vi "PicoScope6000aExampleRapidBlockBulkOverlapped.vi"() -> ()   [LabVIEW 2010]
uses:
  shared/PicoBuffers.ctl
  <vilib>/Waveform/DWDTOps.llb/DWDT Analog to Digital.vi
  PicoScope6000aLib/PicoScope6000aDigitalChannelSettings.ctl
  PicoScope6000aLib/PicoScope6000aAnalogChannelSettings.ctl
  shared/Buffer and Transfer Settings.ctl
  shared/Acquisition Settings.ctl
  shared/Segment Range.ctl
panel:
  in  "Channels":T1={"Channel A Settings "={"Enabled"=TRUE, "Coupling"=50, "Range"=5, "Analogue Offset"=0.0, "BandWidth"=0}, "Channel B Settings "={"Enabled"=FALSE, "Coupling"=50, "Range"=5, "Analogue Offset"=0.0, "BandWidth"=0}, "Channel C Settings "={"Enabled"=FALSE, "Coupling"=50, "Range"=5, "Analogue Offset"=0.0, "BandWidth"=0}, "Channel D Settings "={"Enabled"=FALSE, "Coupling"=50, "Range"=5, "Analogue Offset"=0.0, "BandWidth"=0}, "Channel E Settings "={"Enabled"=FALSE, "Coupling"=50, "Range"=5, "Analogue Offset"=0.0, "BandWidth"=0}, "Channel F Settings "={"Enabled"=FALSE, "Coupling"=50, "Range"=5, "Analogue Offset"=0.0, "BandWidth"=0}, "Channel G Settings "={"Enabled"=FALSE, "Coupling"=50, "Range"=5, "Analogue Offset"=0.0, "BandWidth"=0}, "Channel H Settings "={"Enabled"=FALSE, "Coupling"=50, "Range"=5, "Analogue Offset"=0.0, "BandWidth"=0}} {"Channel H Settings"."BandWidth" items=["Full"=0, "100kHz"=100000, "20kHz"=200000, "1MHz"=1000000, "20MHz"=20000000, "25MHz"=25000000, "50MHz"=50000000, "200MHz"=200000000, "250MHz"=250000000, "500MHz"=500000000]; "Channel H Settings"."Range" items=["10mV"=0, "20mV"=1, "50mV"=2, "100mV"=3, "200mV"=4, "500mV"=5, "1V"=6, "2V"=7, "5V"=8, "10V"=9, "20V"=10, "50V"=11, "100V"=12, "200V"=13, "x10_Probe_100mV"=32, "x10_Probe_200mV"=33, "x10_Probe_500mV"=34, "x10_Probe_1V"=35, "x10_Probe_2V"=36, "x10_Probe_5V"=37, "x10_Probe_10V"=38, "x10_Probe_20V"=39, "x10_Probe_50V"=40, "x10_Probe_100V"=41, "x10_Probe_200V"=42, "x10_Probe_500V"=43, "CURRENT_CLAMP_60A_2A"=10500, "CURRENT_CLAMP_60A_5A"=10501, "CURRENT_CLAMP_60A_10A"=10502, "CURRENT_CLAMP_60A_20A"=10503, "CURRENT_CLAMP_60A_50A"=10504, "CURRENT_CLAMP_60A_60A"=10505, "CURRENT_CLAMP_60A_V2_0_5A"=10600, "CURRENT_CLAMP_60A_V2_1A"=10601, "CURRENT_CLAMP_60A_V2_2A"=10602, "CURRENT_CLAMP_60A_V2_5A"=10603, "CURRENT_CLAMP_60A_V2_10A"=10604, "CURRENT_CLAMP_60A_V2_20A"=10605, "CURRENT_CLAMP_60A_V2_50A"=10606, "CURRENT_CLAMP_60A_V2_60A"=10607, "RESISTANCE_LEAD_NEG5_TO_20OHM"=7000, "RESISTANCE_LEAD_NEG50_TO_200OHM"=7001, "RESISTANCE_LEAD_NEG500_TO_2KOHM"=7002, "RESISTANCE_LEAD_NEG5K_TO_20KOHM"=7003, "RESISTANCE_LEAD_NEG50K_TO_LEAD_200KOHM"=7004, "RESISTANCE_LEAD_NEG500K_TO_LEAD_2MOHM"=7005, "RESISTANCE_LEAD_DIODE_TEST"=7006, "HT_NEG3_TO_5KV"=8950, "HT_NEG3_TO_10KV"=8951, "HT_NEG5_TO_20KV"=8952, "HT_NEG5_TO_50KV"=8953, "HT_NEG5_TO_100KV"=8954, "HT_NEG3_TO_5KV_INVERTED"=8955, "HT_NEG3_TO_10KV_INVERTED"=8956, "HT_NEG5_TO_20KV_INVERTED"=8957, "HT_NEG5_TO_50KV_INVERTED"=8958, "HT_NEG5_TO_100KV_INVERTED"=8959, "TEMPERATURE_NEG50_TO_150DEGC"=9000, "PRESSURE_SENSOR_-100k-150k_PASCALS"=9100, "PRESSURE_SENSOR_-100k_TO_400k_PASCALS"=9101, "PRESSURE_SENSOR_-200k_TO_800k_PASCALS"=9102, "PRESSURE_SENSOR_-400k_TO_1600k_PASCALS"=9103, "PRESSURE_SENSOR_-400k_TO_3400k_PASCALS"=9104, "PRESSURE_SENSOR_-150k_TO_1350k_PASCALS"=9105]; "Channel H Settings"."Coupling" items=["AC"=0, "DC 1M Ohm"=1, "DC 50 Ohm"=50]; "Channel G Settings"."BandWidth" items=["Full"=0, "100kHz"=100000, "20kHz"=200000, "1MHz"=1000000, "20MHz"=20000000, "25MHz"=25000000, "50MHz"=50000000, "200MHz"=200000000, "250MHz"=250000000, "500MHz"=500000000]; "Channel G Settings"."Range" items=["10mV"=0, "20mV"=1, "50mV"=2, "100mV"=3, "200mV"=4, "500mV"=5, "1V"=6, "2V"=7, "5V"=8, "10V"=9, "20V"=10, "50V"=11, "100V"=12, "200V"=13, "x10_Probe_100mV"=32, "x10_Probe_200mV"=33, "x10_Probe_500mV"=34, "x10_Probe_1V"=35, "x10_Probe_2V"=36, "x10_Probe_5V"=37, "x10_Probe_10V"=38, "x10_Probe_20V"=39, "x10_Probe_50V"=40, "x10_Probe_100V"=41, "x10_Probe_200V"=42, "x10_Probe_500V"=43, "CURRENT_CLAMP_60A_2A"=10500, "CURRENT_CLAMP_60A_5A"=10501, "CURRENT_CLAMP_60A_10A"=10502, "CURRENT_CLAMP_60A_20A"=10503, "CURRENT_CLAMP_60A_50A"=10504, "CURRENT_CLAMP_60A_60A"=10505, "CURRENT_CLAMP_60A_V2_0_5A"=10600, "CURRENT_CLAMP_60A_V2_1A"=10601, "CURRENT_CLAMP_60A_V2_2A"=10602, "CURRENT_CLAMP_60A_V2_5A"=10603, "CURRENT_CLAMP_60A_V2_10A"=10604, "CURRENT_CLAMP_60A_V2_20A"=10605, "CURRENT_CLAMP_60A_V2_50A"=10606, "CURRENT_CLAMP_60A_V2_60A"=10607, "RESISTANCE_LEAD_NEG5_TO_20OHM"=7000, "RESISTANCE_LEAD_NEG50_TO_200OHM"=7001, "RESISTANCE_LEAD_NEG500_TO_2KOHM"=7002, "RESISTANCE_LEAD_NEG5K_TO_20KOHM"=7003, "RESISTANCE_LEAD_NEG50K_TO_LEAD_200KOHM"=7004, "RESISTANCE_LEAD_NEG500K_TO_LEAD_2MOHM"=7005, "RESISTANCE_LEAD_DIODE_TEST"=7006, "HT_NEG3_TO_5KV"=8950, "HT_NEG3_TO_10KV"=8951, "HT_NEG5_TO_20KV"=8952, "HT_NEG5_TO_50KV"=8953, "HT_NEG5_TO_100KV"=8954, "HT_NEG3_TO_5KV_INVERTED"=8955, "HT_NEG3_TO_10KV_INVERTED"=8956, "HT_NEG5_TO_20KV_INVERTED"=8957, "HT_NEG5_TO_50KV_INVERTED"=8958, "HT_NEG5_TO_100KV_INVERTED"=8959, "TEMPERATURE_NEG50_TO_150DEGC"=9000, "PRESSURE_SENSOR_-100k-150k_PASCALS"=9100, "PRESSURE_SENSOR_-100k_TO_400k_PASCALS"=9101, "PRESSURE_SENSOR_-200k_TO_800k_PASCALS"=9102, "PRESSURE_SENSOR_-400k_TO_1600k_PASCALS"=9103, "PRESSURE_SENSOR_-400k_TO_3400k_PASCALS"=9104, "PRESSURE_SENSOR_-150k_TO_1350k_PASCALS"=9105]; "Channel G Settings"."Coupling" items=["AC"=0, "DC 1M Ohm"=1, "DC 50 Ohm"=50]; "Channel F Settings"."BandWidth" items=["Full"=0, "100kHz"=100000, "20kHz"=200000, "1MHz"=1000000, "20MHz"=20000000, "25MHz"=25000000, "50MHz"=50000000, "200MHz"=200000000, "250MHz"=250000000, "500MHz"=500000000]; "Channel F Settings"."Range" items=["10mV"=0, "20mV"=1, "50mV"=2, "100mV"=3, "200mV"=4, "500mV"=5, "1V"=6, "2V"=7, "5V"=8, "10V"=9, "20V"=10, "50V"=11, "100V"=12, "200V"=13, "x10_Probe_100mV"=32, "x10_Probe_200mV"=33, "x10_Probe_500mV"=34, "x10_Probe_1V"=35, "x10_Probe_2V"=36, "x10_Probe_5V"=37, "x10_Probe_10V"=38, "x10_Probe_20V"=39, "x10_Probe_50V"=40, "x10_Probe_100V"=41, "x10_Probe_200V"=42, "x10_Probe_500V"=43, "CURRENT_CLAMP_60A_2A"=10500, "CURRENT_CLAMP_60A_5A"=10501, "CURRENT_CLAMP_60A_10A"=10502, "CURRENT_CLAMP_60A_20A"=10503, "CURRENT_CLAMP_60A_50A"=10504, "CURRENT_CLAMP_60A_60A"=10505, "CURRENT_CLAMP_60A_V2_0_5A"=10600, "CURRENT_CLAMP_60A_V2_1A"=10601, "CURRENT_CLAMP_60A_V2_2A"=10602, "CURRENT_CLAMP_60A_V2_5A"=10603, "CURRENT_CLAMP_60A_V2_10A"=10604, "CURRENT_CLAMP_60A_V2_20A"=10605, "CURRENT_CLAMP_60A_V2_50A"=10606, "CURRENT_CLAMP_60A_V2_60A"=10607, "RESISTANCE_LEAD_NEG5_TO_20OHM"=7000, "RESISTANCE_LEAD_NEG50_TO_200OHM"=7001, "RESISTANCE_LEAD_NEG500_TO_2KOHM"=7002, "RESISTANCE_LEAD_NEG5K_TO_20KOHM"=7003, "RESISTANCE_LEAD_NEG50K_TO_LEAD_200KOHM"=7004, "RESISTANCE_LEAD_NEG500K_TO_LEAD_2MOHM"=7005, "RESISTANCE_LEAD_DIODE_TEST"=7006, "HT_NEG3_TO_5KV"=8950, "HT_NEG3_TO_10KV"=8951, "HT_NEG5_TO_20KV"=8952, "HT_NEG5_TO_50KV"=8953, "HT_NEG5_TO_100KV"=8954, "HT_NEG3_TO_5KV_INVERTED"=8955, "HT_NEG3_TO_10KV_INVERTED"=8956, "HT_NEG5_TO_20KV_INVERTED"=8957, "HT_NEG5_TO_50KV_INVERTED"=8958, "HT_NEG5_TO_100KV_INVERTED"=8959, "TEMPERATURE_NEG50_TO_150DEGC"=9000, "PRESSURE_SENSOR_-100k-150k_PASCALS"=9100, "PRESSURE_SENSOR_-100k_TO_400k_PASCALS"=9101, "PRESSURE_SENSOR_-200k_TO_800k_PASCALS"=9102, "PRESSURE_SENSOR_-400k_TO_1600k_PASCALS"=9103, "PRESSURE_SENSOR_-400k_TO_3400k_PASCALS"=9104, "PRESSURE_SENSOR_-150k_TO_1350k_PASCALS"=9105]; "Channel F Settings"."Coupling" items=["AC"=0, "DC 1M Ohm"=1, "DC 50 Ohm"=50]; "Channel E Settings"."BandWidth" items=["Full"=0, "100kHz"=100000, "20kHz"=200000, "1MHz"=1000000, "20MHz"=20000000, "25MHz"=25000000, "50MHz"=50000000, "200MHz"=200000000, "250MHz"=250000000, "500MHz"=500000000]; "Channel E Settings"."Range" items=["10mV"=0, "20mV"=1, "50mV"=2, "100mV"=3, "200mV"=4, "500mV"=5, "1V"=6, "2V"=7, "5V"=8, "10V"=9, "20V"=10, "50V"=11, "100V"=12, "200V"=13, "x10_Probe_100mV"=32, "x10_Probe_200mV"=33, "x10_Probe_500mV"=34, "x10_Probe_1V"=35, "x10_Probe_2V"=36, "x10_Probe_5V"=37, "x10_Probe_10V"=38, "x10_Probe_20V"=39, "x10_Probe_50V"=40, "x10_Probe_100V"=41, "x10_Probe_200V"=42, "x10_Probe_500V"=43, "CURRENT_CLAMP_60A_2A"=10500, "CURRENT_CLAMP_60A_5A"=10501, "CURRENT_CLAMP_60A_10A"=10502, "CURRENT_CLAMP_60A_20A"=10503, "CURRENT_CLAMP_60A_50A"=10504, "CURRENT_CLAMP_60A_60A"=10505, "CURRENT_CLAMP_60A_V2_0_5A"=10600, "CURRENT_CLAMP_60A_V2_1A"=10601, "CURRENT_CLAMP_60A_V2_2A"=10602, "CURRENT_CLAMP_60A_V2_5A"=10603, "CURRENT_CLAMP_60A_V2_10A"=10604, "CURRENT_CLAMP_60A_V2_20A"=10605, "CURRENT_CLAMP_60A_V2_50A"=10606, "CURRENT_CLAMP_60A_V2_60A"=10607, "RESISTANCE_LEAD_NEG5_TO_20OHM"=7000, "RESISTANCE_LEAD_NEG50_TO_200OHM"=7001, "RESISTANCE_LEAD_NEG500_TO_2KOHM"=7002, "RESISTANCE_LEAD_NEG5K_TO_20KOHM"=7003, "RESISTANCE_LEAD_NEG50K_TO_LEAD_200KOHM"=7004, "RESISTANCE_LEAD_NEG500K_TO_LEAD_2MOHM"=7005, "RESISTANCE_LEAD_DIODE_TEST"=7006, "HT_NEG3_TO_5KV"=8950, "HT_NEG3_TO_10KV"=8951, "HT_NEG5_TO_20KV"=8952, "HT_NEG5_TO_50KV"=8953, "HT_NEG5_TO_100KV"=8954, "HT_NEG3_TO_5KV_INVERTED"=8955, "HT_NEG3_TO_10KV_INVERTED"=8956, "HT_NEG5_TO_20KV_INVERTED"=8957, "HT_NEG5_TO_50KV_INVERTED"=8958, "HT_NEG5_TO_100KV_INVERTED"=8959, "TEMPERATURE_NEG50_TO_150DEGC"=9000, "PRESSURE_SENSOR_-100k-150k_PASCALS"=9100, "PRESSURE_SENSOR_-100k_TO_400k_PASCALS"=9101, "PRESSURE_SENSOR_-200k_TO_800k_PASCALS"=9102, "PRESSURE_SENSOR_-400k_TO_1600k_PASCALS"=9103, "PRESSURE_SENSOR_-400k_TO_3400k_PASCALS"=9104, "PRESSURE_SENSOR_-150k_TO_1350k_PASCALS"=9105]; "Channel E Settings"."Coupling" items=["AC"=0, "DC 1M Ohm"=1, "DC 50 Ohm"=50]; "Channel D Settings"."BandWidth" items=["Full"=0, "100kHz"=100000, "20kHz"=200000, "1MHz"=1000000, "20MHz"=20000000, "25MHz"=25000000, "50MHz"=50000000, "200MHz"=200000000, "250MHz"=250000000, "500MHz"=500000000]; "Channel D Settings"."Range" items=["10mV"=0, "20mV"=1, "50mV"=2, "100mV"=3, "200mV"=4, "500mV"=5, "1V"=6, "2V"=7, "5V"=8, "10V"=9, "20V"=10, "50V"=11, "100V"=12, "200V"=13, "x10_Probe_100mV"=32, "x10_Probe_200mV"=33, "x10_Probe_500mV"=34, "x10_Probe_1V"=35, "x10_Probe_2V"=36, "x10_Probe_5V"=37, "x10_Probe_10V"=38, "x10_Probe_20V"=39, "x10_Probe_50V"=40, "x10_Probe_100V"=41, "x10_Probe_200V"=42, "x10_Probe_500V"=43, "CURRENT_CLAMP_60A_2A"=10500, "CURRENT_CLAMP_60A_5A"=10501, "CURRENT_CLAMP_60A_10A"=10502, "CURRENT_CLAMP_60A_20A"=10503, "CURRENT_CLAMP_60A_50A"=10504, "CURRENT_CLAMP_60A_60A"=10505, "CURRENT_CLAMP_60A_V2_0_5A"=10600, "CURRENT_CLAMP_60A_V2_1A"=10601, "CURRENT_CLAMP_60A_V2_2A"=10602, "CURRENT_CLAMP_60A_V2_5A"=10603, "CURRENT_CLAMP_60A_V2_10A"=10604, "CURRENT_CLAMP_60A_V2_20A"=10605, "CURRENT_CLAMP_60A_V2_50A"=10606, "CURRENT_CLAMP_60A_V2_60A"=10607, "RESISTANCE_LEAD_NEG5_TO_20OHM"=7000, "RESISTANCE_LEAD_NEG50_TO_200OHM"=7001, "RESISTANCE_LEAD_NEG500_TO_2KOHM"=7002, "RESISTANCE_LEAD_NEG5K_TO_20KOHM"=7003, "RESISTANCE_LEAD_NEG50K_TO_LEAD_200KOHM"=7004, "RESISTANCE_LEAD_NEG500K_TO_LEAD_2MOHM"=7005, "RESISTANCE_LEAD_DIODE_TEST"=7006, "HT_NEG3_TO_5KV"=8950, "HT_NEG3_TO_10KV"=8951, "HT_NEG5_TO_20KV"=8952, "HT_NEG5_TO_50KV"=8953, "HT_NEG5_TO_100KV"=8954, "HT_NEG3_TO_5KV_INVERTED"=8955, "HT_NEG3_TO_10KV_INVERTED"=8956, "HT_NEG5_TO_20KV_INVERTED"=8957, "HT_NEG5_TO_50KV_INVERTED"=8958, "HT_NEG5_TO_100KV_INVERTED"=8959, "TEMPERATURE_NEG50_TO_150DEGC"=9000, "PRESSURE_SENSOR_-100k-150k_PASCALS"=9100, "PRESSURE_SENSOR_-100k_TO_400k_PASCALS"=9101, "PRESSURE_SENSOR_-200k_TO_800k_PASCALS"=9102, "PRESSURE_SENSOR_-400k_TO_1600k_PASCALS"=9103, "PRESSURE_SENSOR_-400k_TO_3400k_PASCALS"=9104, "PRESSURE_SENSOR_-150k_TO_1350k_PASCALS"=9105]; "Channel D Settings"."Coupling" items=["AC"=0, "DC 1M Ohm"=1, "DC 50 Ohm"=50]; "Channel C Settings"."BandWidth" items=["Full"=0, "100kHz"=100000, "20kHz"=200000, "1MHz"=1000000, "20MHz"=20000000, "25MHz"=25000000, "50MHz"=50000000, "200MHz"=200000000, "250MHz"=250000000, "500MHz"=500000000]; "Channel C Settings"."Range" items=["10mV"=0, "20mV"=1, "50mV"=2, "100mV"=3, "200mV"=4, "500mV"=5, "1V"=6, "2V"=7, "5V"=8, "10V"=9, "20V"=10, "50V"=11, "100V"=12, "200V"=13, "x10_Probe_100mV"=32, "x10_Probe_200mV"=33, "x10_Probe_500mV"=34, "x10_Probe_1V"=35, "x10_Probe_2V"=36, "x10_Probe_5V"=37, "x10_Probe_10V"=38, "x10_Probe_20V"=39, "x10_Probe_50V"=40, "x10_Probe_100V"=41, "x10_Probe_200V"=42, "x10_Probe_500V"=43, "CURRENT_CLAMP_60A_2A"=10500, "CURRENT_CLAMP_60A_5A"=10501, "CURRENT_CLAMP_60A_10A"=10502, "CURRENT_CLAMP_60A_20A"=10503, "CURRENT_CLAMP_60A_50A"=10504, "CURRENT_CLAMP_60A_60A"=10505, "CURRENT_CLAMP_60A_V2_0_5A"=10600, "CURRENT_CLAMP_60A_V2_1A"=10601, "CURRENT_CLAMP_60A_V2_2A"=10602, "CURRENT_CLAMP_60A_V2_5A"=10603, "CURRENT_CLAMP_60A_V2_10A"=10604, "CURRENT_CLAMP_60A_V2_20A"=10605, "CURRENT_CLAMP_60A_V2_50A"=10606, "CURRENT_CLAMP_60A_V2_60A"=10607, "RESISTANCE_LEAD_NEG5_TO_20OHM"=7000, "RESISTANCE_LEAD_NEG50_TO_200OHM"=7001, "RESISTANCE_LEAD_NEG500_TO_2KOHM"=7002, "RESISTANCE_LEAD_NEG5K_TO_20KOHM"=7003, "RESISTANCE_LEAD_NEG50K_TO_LEAD_200KOHM"=7004, "RESISTANCE_LEAD_NEG500K_TO_LEAD_2MOHM"=7005, "RESISTANCE_LEAD_DIODE_TEST"=7006, "HT_NEG3_TO_5KV"=8950, "HT_NEG3_TO_10KV"=8951, "HT_NEG5_TO_20KV"=8952, "HT_NEG5_TO_50KV"=8953, "HT_NEG5_TO_100KV"=8954, "HT_NEG3_TO_5KV_INVERTED"=8955, "HT_NEG3_TO_10KV_INVERTED"=8956, "HT_NEG5_TO_20KV_INVERTED"=8957, "HT_NEG5_TO_50KV_INVERTED"=8958, "HT_NEG5_TO_100KV_INVERTED"=8959, "TEMPERATURE_NEG50_TO_150DEGC"=9000, "PRESSURE_SENSOR_-100k-150k_PASCALS"=9100, "PRESSURE_SENSOR_-100k_TO_400k_PASCALS"=9101, "PRESSURE_SENSOR_-200k_TO_800k_PASCALS"=9102, "PRESSURE_SENSOR_-400k_TO_1600k_PASCALS"=9103, "PRESSURE_SENSOR_-400k_TO_3400k_PASCALS"=9104, "PRESSURE_SENSOR_-150k_TO_1350k_PASCALS"=9105]; "Channel C Settings"."Coupling" items=["AC"=0, "DC 1M Ohm"=1, "DC 50 Ohm"=50]; "Channel B Settings"."BandWidth" items=["Full"=0, "100kHz"=100000, "20kHz"=200000, "1MHz"=1000000, "20MHz"=20000000, "25MHz"=25000000, "50MHz"=50000000, "200MHz"=200000000, "250MHz"=250000000, "500MHz"=500000000]; "Channel B Settings"."Range" items=["10mV"=0, "20mV"=1, "50mV"=2, "100mV"=3, "200mV"=4, "500mV"=5, "1V"=6, "2V"=7, "5V"=8, "10V"=9, "20V"=10, "50V"=11, "100V"=12, "200V"=13, "x10_Probe_100mV"=32, "x10_Probe_200mV"=33, "x10_Probe_500mV"=34, "x10_Probe_1V"=35, "x10_Probe_2V"=36, "x10_Probe_5V"=37, "x10_Probe_10V"=38, "x10_Probe_20V"=39, "x10_Probe_50V"=40, "x10_Probe_100V"=41, "x10_Probe_200V"=42, "x10_Probe_500V"=43, "CURRENT_CLAMP_60A_2A"=10500, "CURRENT_CLAMP_60A_5A"=10501, "CURRENT_CLAMP_60A_10A"=10502, "CURRENT_CLAMP_60A_20A"=10503, "CURRENT_CLAMP_60A_50A"=10504, "CURRENT_CLAMP_60A_60A"=10505, "CURRENT_CLAMP_60A_V2_0_5A"=10600, "CURRENT_CLAMP_60A_V2_1A"=10601, "CURRENT_CLAMP_60A_V2_2A"=10602, "CURRENT_CLAMP_60A_V2_5A"=10603, "CURRENT_CLAMP_60A_V2_10A"=10604, "CURRENT_CLAMP_60A_V2_20A"=10605, "CURRENT_CLAMP_60A_V2_50A"=10606, "CURRENT_CLAMP_60A_V2_60A"=10607, "RESISTANCE_LEAD_NEG5_TO_20OHM"=7000, "RESISTANCE_LEAD_NEG50_TO_200OHM"=7001, "RESISTANCE_LEAD_NEG500_TO_2KOHM"=7002, "RESISTANCE_LEAD_NEG5K_TO_20KOHM"=7003, "RESISTANCE_LEAD_NEG50K_TO_LEAD_200KOHM"=7004, "RESISTANCE_LEAD_NEG500K_TO_LEAD_2MOHM"=7005, "RESISTANCE_LEAD_DIODE_TEST"=7006, "HT_NEG3_TO_5KV"=8950, "HT_NEG3_TO_10KV"=8951, "HT_NEG5_TO_20KV"=8952, "HT_NEG5_TO_50KV"=8953, "HT_NEG5_TO_100KV"=8954, "HT_NEG3_TO_5KV_INVERTED"=8955, "HT_NEG3_TO_10KV_INVERTED"=8956, "HT_NEG5_TO_20KV_INVERTED"=8957, "HT_NEG5_TO_50KV_INVERTED"=8958, "HT_NEG5_TO_100KV_INVERTED"=8959, "TEMPERATURE_NEG50_TO_150DEGC"=9000, "PRESSURE_SENSOR_-100k-150k_PASCALS"=9100, "PRESSURE_SENSOR_-100k_TO_400k_PASCALS"=9101, "PRESSURE_SENSOR_-200k_TO_800k_PASCALS"=9102, "PRESSURE_SENSOR_-400k_TO_1600k_PASCALS"=9103, "PRESSURE_SENSOR_-400k_TO_3400k_PASCALS"=9104, "PRESSURE_SENSOR_-150k_TO_1350k_PASCALS"=9105]; "Channel B Settings"."Coupling" items=["AC"=0, "DC 1M Ohm"=1, "DC 50 Ohm"=50]; "Channel A Settings"."Range" items=["10mV"=0, "20mV"=1, "50mV"=2, "100mV"=3, "200mV"=4, "500mV"=5, "1V"=6, "2V"=7, "5V"=8, "10V"=9, "20V"=10, "50V"=11, "100V"=12, "200V"=13, "x10_Probe_100mV"=32, "x10_Probe_200mV"=33, "x10_Probe_500mV"=34, "x10_Probe_1V"=35, "x10_Probe_2V"=36, "x10_Probe_5V"=37, "x10_Probe_10V"=38, "x10_Probe_20V"=39, "x10_Probe_50V"=40, "x10_Probe_100V"=41, "x10_Probe_200V"=42, "x10_Probe_500V"=43, "CURRENT_CLAMP_60A_2A"=10500, "CURRENT_CLAMP_60A_5A"=10501, "CURRENT_CLAMP_60A_10A"=10502, "CURRENT_CLAMP_60A_20A"=10503, "CURRENT_CLAMP_60A_50A"=10504, "CURRENT_CLAMP_60A_60A"=10505, "CURRENT_CLAMP_60A_V2_0_5A"=10600, "CURRENT_CLAMP_60A_V2_1A"=10601, "CURRENT_CLAMP_60A_V2_2A"=10602, "CURRENT_CLAMP_60A_V2_5A"=10603, "CURRENT_CLAMP_60A_V2_10A"=10604, "CURRENT_CLAMP_60A_V2_20A"=10605, "CURRENT_CLAMP_60A_V2_50A"=10606, "CURRENT_CLAMP_60A_V2_60A"=10607, "RESISTANCE_LEAD_NEG5_TO_20OHM"=7000, "RESISTANCE_LEAD_NEG50_TO_200OHM"=7001, "RESISTANCE_LEAD_NEG500_TO_2KOHM"=7002, "RESISTANCE_LEAD_NEG5K_TO_20KOHM"=7003, "RESISTANCE_LEAD_NEG50K_TO_LEAD_200KOHM"=7004, "RESISTANCE_LEAD_NEG500K_TO_LEAD_2MOHM"=7005, "RESISTANCE_LEAD_DIODE_TEST"=7006, "HT_NEG3_TO_5KV"=8950, "HT_NEG3_TO_10KV"=8951, "HT_NEG5_TO_20KV"=8952, "HT_NEG5_TO_50KV"=8953, "HT_NEG5_TO_100KV"=8954, "HT_NEG3_TO_5KV_INVERTED"=8955, "HT_NEG3_TO_10KV_INVERTED"=8956, "HT_NEG5_TO_20KV_INVERTED"=8957, "HT_NEG5_TO_50KV_INVERTED"=8958, "HT_NEG5_TO_100KV_INVERTED"=8959, "TEMPERATURE_NEG50_TO_150DEGC"=9000, "PRESSURE_SENSOR_-100k-150k_PASCALS"=9100, "PRESSURE_SENSOR_-100k_TO_400k_PASCALS"=9101, "PRESSURE_SENSOR_-200k_TO_800k_PASCALS"=9102, "PRESSURE_SENSOR_-400k_TO_1600k_PASCALS"=9103, "PRESSURE_SENSOR_-400k_TO_3400k_PASCALS"=9104, "PRESSURE_SENSOR_-150k_TO_1350k_PASCALS"=9105]; "Channel A Settings"."BandWidth" items=["Full"=0, "100kHz"=100000, "20kHz"=200000, "1MHz"=1000000, "20MHz"=20000000, "25MHz"=25000000, "50MHz"=50000000, "200MHz"=200000000, "250MHz"=250000000, "500MHz"=500000000]; "Channel A Settings"."Coupling" items=["AC"=0, "DC 1M Ohm"=1, "DC 50 Ohm"=50]}
  out "overflow":i16[](array[numeric])=[1023] format="%010d"
  out "Trigger Offsets":cluster{"Samples":u64, "Time (seconds)":sgl}[](array[cluster]) {"Time (seconds)" format="%#_5p"}
  in  "Stop Display":bool
  out "Capture Complete":bool
  in  "Run":bool
  in  "Display Buffer Index":i32
  in  "Segment Range":T2={"fromSegmentIndex"=0, "toSegmentIndex"=9} {"toSegmentIndex" format="%.4p"; "fromSegmentIndex" format="%.4p"}
  in  "nSegments":u64=10 format="%.4p"
  out "error out":errorcluster
  in  "Data file":path=path "PicoScope6000aExampleRapidBlock ChA Data"
  in  "Digital Channels":T3={"Port 0 Settings "={"Enabled"=FALSE, "Hysteresis"=3, "Threshold Level (Volts)"=[1.0, 1.0, 1.0, 1.0, 1.0, 1.0, 1.0, 1.0]}, "Port 1 Settings"={"Enabled"=FALSE, "Hysteresis"=3, "Threshold Level (Volts)"=[1.0, 1.0, 1.0, 1.0, 1.0, 1.0, 1.0, 1.0]}} {"Port 1 Settings"."Threshold Level (Volts)" format="%#_4p"; "Port 1 Settings"."Hysteresis" items=["PICO_VERY_HIGH_400MV", "PICO_HIGH_200MV", "PICO_NORMAL_100MV", "PICO_LOW_50MV"]; "Port 0 Settings"."Threshold Level (Volts)" format="%#_4p"; "Port 0 Settings"."Hysteresis" items=["PICO_VERY_HIGH_400MV", "PICO_HIGH_200MV", "PICO_NORMAL_100MV", "PICO_LOW_50MV"]}
  in  "Trigger Settings":T4={"Trigger Enabled"=FALSE, "Trigger Threshold (Volts)"=0.0, "Trigger Direction"=2, "Trigger Delay (samples)"=0, "Auto Trigger Time (us)"=1000000, "Trigger Source"=0} {"Trigger Source" items=["Channel A"=0, "Channel B"=1, "Channel C"=2, "Channel D"=3, "Channel E"=4, "Channel F"=5, "Channel G"=6, "Channel H"=7, "Port 0"=128, "Port 1"=129, "Trigger AUX"=1001]; "Auto Trigger Time (us)" format="%.4p"; "Trigger Direction" items=["Above", "Below", "Rising", "Falling", "Rising or Falling"]; "Trigger Threshold (Volts)" format="%#_6p"}
  in  "Buffer and Transfer Settings":T5={"startIndex"=0, "Samples"=10000000, "Down Sample Ratio"=16, "Down-Sample Mode"=1} {"Down-Sample Mode" items=["RAW none"=2147483648, "None"=0, "Aggregate"=1, "Decimate"=2, "Average"=4]; "Down Sample Ratio" step=1; "Samples" format="%_6p"}
  in  "Acquisition Settings":T6={"preTriggerSamples"=0, "postTriggerSamples"=10000000, "timebase"=5} {"postTriggerSamples" format="%_6p"; "preTriggerSamples" format="%_6p"}
  out "Properties Panel":T7 {"Max Total Capture Time Available (sec)" format="%.3p"; "Sample Frequency" format="%.6p"; "Sample Rate" format="%.3p"; "Max Samples Available" format="%_6p"; "Total Capture Time (sec)" format="%.3p"}
  out "Port 0":digitalwaveform(graph)={"t0"=timestamp(0 s since 1904-01-01), "dt"=8e-09, "Y"={"transitions"=[], "data"=[]}}
  in  "stop":bool
  out "Analog Channels":cluster{i32, dbl, "Data":dbl[]}[](graph)
  out "Device Info":T8={"PICO_DRIVER_VERSION"="", "PICO_USB_VERSION"="", "PICO_HARDWARE_VERSION"="", "PICO_VARIANT_INFO"="", "PICO_BATCH_AND_SERIAL"="", "PICO_CAL_DATE"="", "PICO_KERNEL_VERSION"="", "PICO_DIGITAL_HARDWARE_VERSION"="", "PICO_ANALOGUE_HARDWARE_VERSION"="", "PICO_FIRMWARE_VERSION_1"="", "PICO_FIRMWARE_VERSION_2"="", "PICO_IPP_VERSION"="", "PICO_DRIVER_PATH"="", "PICO_FIRMWARE_VERSION_3"="", "PICO_FRONT_PANEL_FIRMWARE_VERSION"="", "Number of Channels"=8, "MSO"=FALSE}
  out "Pico 6000a Units":string
  in  "Resolution":u32(ring) items=["8-bit"=0, "12-bit"=1, "14-bit"=2, "15-bit"=3, "16-bit"=4, "10-bit"=10]
  in  "Serial Number":string
  in  "Use Serial Number":bool
  in  "error in (no error)":errorcluster
  # "Please Ensure you set the \"Range\"(Probe type) before running the VI"
  # "Bit 0 = ChA"
  # "D8-D15"
  # "DO-D7"
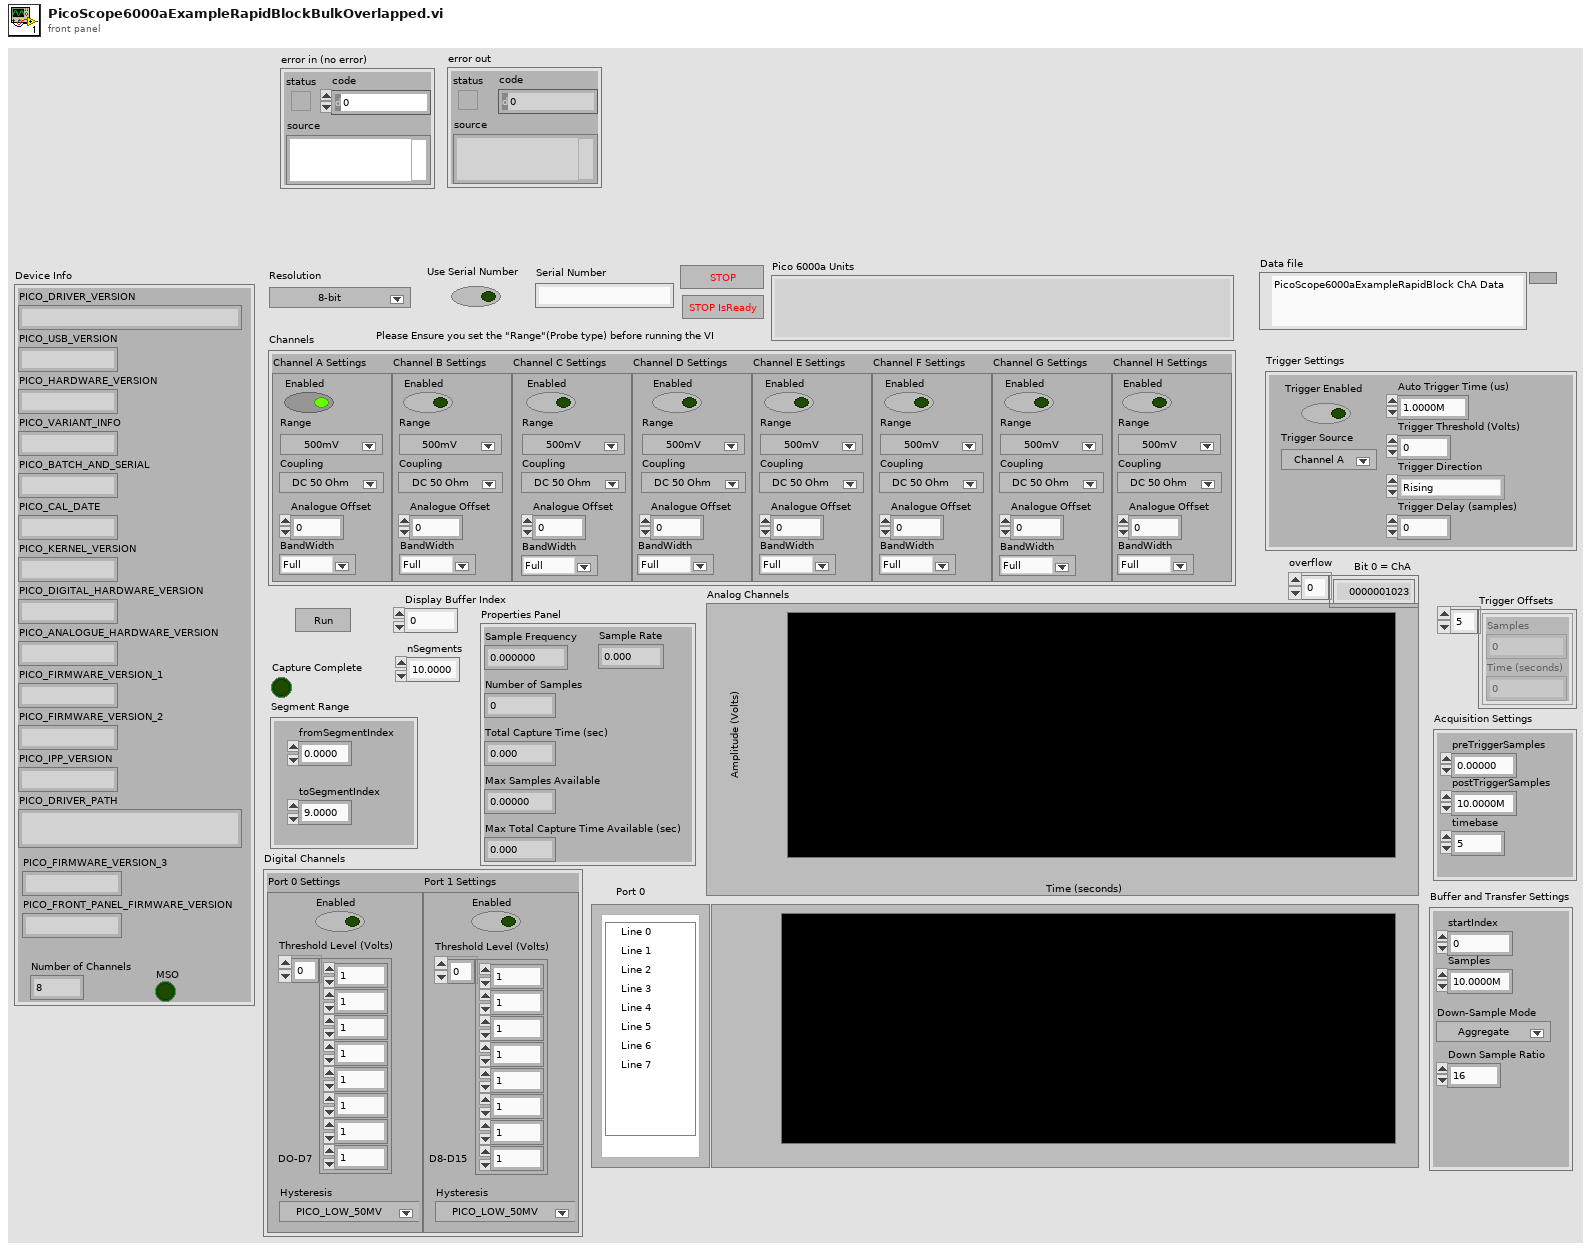
[diagram p1: front panel]
types:
  T1 = typedef "PicoScope6000aAnalogChannelSettings.ctl" = cluster{"Channel A Settings ":cluster{"Enabled":bool, "Coupling":i16, "Range":u16, "Analogue Offset":dbl, "BandWidth":u32}, "Channel B Settings ":cluster{"Enabled":bool, "Coupling":i16, "Range":u16, "Analogue Offset":dbl, "BandWidth":u32}, "Channel C Settings ":cluster{"Enabled":bool, "Coupling":i16, "Range":u16, "Analogue Offset":dbl, "BandWidth":u32}, "Channel D Settings ":cluster{"Enabled":bool, "Coupling":i16, "Range":u16, "Analogue Offset":dbl, "BandWidth":u32}, "Channel E Settings ":cluster{"Enabled":bool, "Coupling":i16, "Range":u16, "Analogue Offset":dbl, "BandWidth":u32}, "Channel F Settings ":cluster{"Enabled":bool, "Coupling":i16, "Range":u16, "Analogue Offset":dbl, "BandWidth":u32}, "Channel G Settings ":cluster{"Enabled":bool, "Coupling":i16, "Range":u16, "Analogue Offset":dbl, "BandWidth":u32}, "Channel H Settings ":cluster{"Enabled":bool, "Coupling":i16, "Range":u16, "Analogue Offset":dbl, "BandWidth":u32}}
  T2 = typedef "Segment Range.ctl" = cluster{"fromSegmentIndex":u64, "toSegmentIndex":u64}
  T3 = typedef "PicoScope6000aDigitalChannelSettings.ctl" = cluster{"Port 0 Settings ":cluster{"Enabled":bool, "Hysteresis":u32, "Threshold Level (Volts)":dbl[]}, "Port 1 Settings":cluster{"Enabled":bool, "Hysteresis":u32, "Threshold Level (Volts)":dbl[]}}
  T4 = cluster{"Trigger Enabled":bool, "Trigger Threshold (Volts)":dbl, "Trigger Direction":u16, "Trigger Delay (samples)":u64, "Auto Trigger Time (us)":u32, "Trigger Source":u32}
  T5 = typedef "Buffer and Transfer Settings.ctl" = cluster{"startIndex":u64, "Samples":u64, "Down Sample Ratio":u64, "Down-Sample Mode":u32}
  T6 = typedef "Acquisition Settings.ctl" = cluster{"preTriggerSamples":u64, "postTriggerSamples":u64, "timebase":u32}
  T7 = cluster{"Sample Frequency":dbl, "Sample Rate":dbl, "Max Samples Available":u64, "Number of Samples":u64, "Total Capture Time (sec) ":dbl, "Max Total Capture Time Available (sec)":dbl}
  T8 = cluster{"PICO_DRIVER_VERSION":string, "PICO_USB_VERSION":string, "PICO_HARDWARE_VERSION":string, "PICO_VARIANT_INFO":string, "PICO_BATCH_AND_SERIAL":string, "PICO_CAL_DATE":string, "PICO_KERNEL_VERSION":string, "PICO_DIGITAL_HARDWARE_VERSION":string, "PICO_ANALOGUE_HARDWARE_VERSION":string, "PICO_FIRMWARE_VERSION_1":string, "PICO_FIRMWARE_VERSION_2":string, "PICO_IPP_VERSION":string, "PICO_DRIVER_PATH":string, "PICO_FIRMWARE_VERSION_3":string, "PICO_FRONT_PANEL_FIRMWARE_VERSION":string, "Number of Channels":i16, "MSO":bool}
  T9 = enum16{"open", "open or create", "create or replace", "create", "open (read-only)"}
  T10 = typedef "PicoBuffers.ctl" = cluster{"Max Buffer Pointers":u64[][][], "Min Buffer Pointers":u64[][][], "StreamingDataInfo":cluster{"Channel":u32, "Down-Sample Mode":u32, "PICO_DATA_TYPE":enum32{"PICO_INT8_T", "PICO_INT16_T", "PICO_INT32_T", "PICO_UINT32_T", "PICO_INT64_T", ""}, "Samples":i32, "bufferIndex":u64, "startIndex":i32, "overflow":i16}[][]}
  T11 = cluster{"Channel A Buffer":i16[], "Channel B Buffer":i16[], "Channel C Buffer":i16[], "Channel D Buffer":i16[], "Channel E Buffer":i16[], "Channel F Buffer":i16[], "Channel G Buffer":i16[], "Channel H Buffer":i16[], "Port 0 Buffer":i16[], "Port 1 Buffer":i16[]}[]
  T12 = cluster{"Channel A Buffer":i16[], "Channel B Buffer":i16[], "Channel C Buffer":i16[], "Channel D Buffer":i16[], "Channel E Buffer":i16[], "Channel F Buffer":i16[], "Channel G Buffer":i16[], "Channel H Buffer":i16[], "Port 0 Buffer":i16[], "Port 1 Buffer":i16[]}
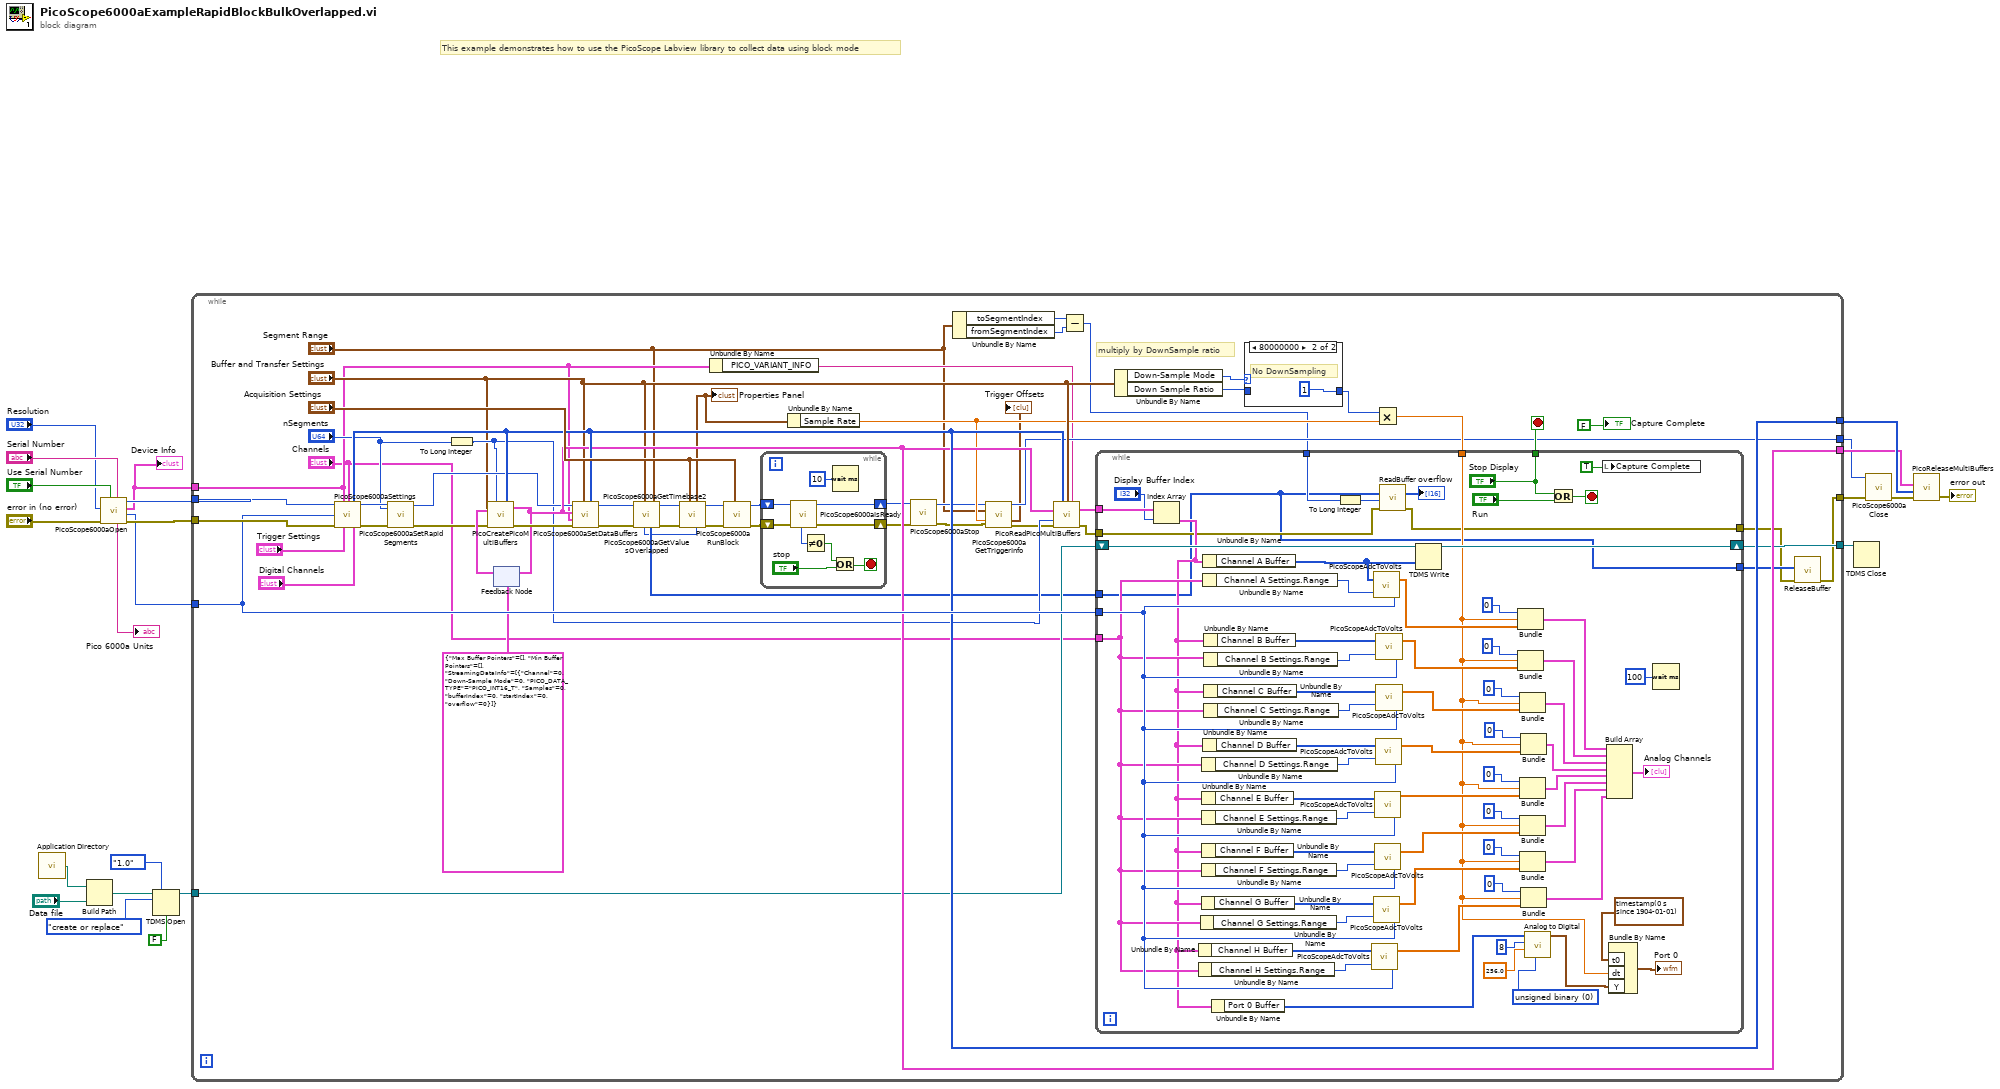
[diagram p0: block diagram]
diagram:
  # "This example demonstrates how to use the PicoScope Labview library to collect data using block mode"
  n1 = call <vilib>:"Application Directory.vi"() -> ("Application Directory"=w4:path)
  n2 = Build Path(base path=w4, name or relative path="Data file") -> (appended path=w5:path)
  n3 = call "PicoScope6000aOpen.vi"("Serial Number"="Serial Number", "Use Serial Number"="Use Serial Number", "error in (no error)"="error in (no error)", "Resolution"="Resolution") -> ("error out"=w19:errorcluster, "Max ADC value"=w16:i16, "Device Info"=w15:T8, "handle out"=w20:i16, "Pico 6000a Units"=→"Pico 6000a Units":string)  [unwired: 2 in, 1 out]
  "Device Info" <- w15
  n4 = TDMS Open(6:FALSE ("disable buffering? (T)"), 7:enum16{"1.0", "2.0"}."1.0" ("file format version (2.0)"), 10:T9."create or replace" ("operation (0:open)"), 11:w5) -> (3:w2:refnum<k34>)  [unwired: 2 in, 1 out]
  n5 = while {
    tunnel: w15 -> [w34]
    tunnel: w16 -> [w78]
    tunnel: w20 -> [w80]
    tunnel: [w42] -> w11
    tunnel: w19 -> [w79]
    tunnel: [w26] -> w12
    tunnel: [w71] -> w14
    tunnel: [w70] -> w13
    tunnel: [w69] -> w3
    tunnel: w2 -> [w68]
    stop <- w48 stop-if-true
    # "multiply by DownSample ratio"
    n6 = call "PicoScope6000aSettings.vi"("handle in"=w80, "Device Info"=w34, "Channels"="Channels", "Max ADC value"=w78, "error in (no error)"=w79, "Trigger Settings"="Trigger Settings", "Digital Channels"="Digital Channels") -> ("Enabled array"=w71:i16[], "handle out"=w66:i16, "error out"=w67:errorcluster)  [unwired: 6 in]
    n7 = call "PicoScope6000aSetRapidSegments.vi"("nSegments"="nSegments", "error in (no error)"=w67, "handle in"=w66) -> ("error out"=w65:errorcluster, "handle out"=w64:i16)  [unwired: 6 in, 1 out]
    n8 = To Long Integer(number="nSegments") -> (32bit integer=w60:i32)
    n9 = feedback #1(T10 {"Max Buffer Pointers"=[], "Min Buffer Pointers"=[], "StreamingDataInfo"=[[{"Channel"=0, "Down-Sample Mode"=0, "PICO_DATA_TYPE"=enum."PICO_INT16_T", "Samples"=0, "bufferIndex"=0, "startIndex"=0, "overflow"=0}]]} ("Data Pointers")) -> (w74:T10)
    n10 = call "PicoCreatePicoMultiBuffers.vi"("Number of Buffers"=w60, "Buffer and Transfer Settings"="Buffer and Transfer Settings", "enabled array"=w71, "Data Pointers In"=w74, "error in (no error)"=w65) -> ("Data Pointers"=w70:T10, "error out"=w72:errorcluster)  [unwired: 9 in]
    n11 = feedback-in #1(w70) -> ()
    n12 = call "PicoScope6000aSetDataBuffers.vi"("enabled array"=w71, "Buffer and Transfer Settings"="Buffer and Transfer Settings", "error in (no error)"=w72, "Device Info"=w34, "Data Pointers In"=w70, "handle in"=w64) -> ("error out"=w63:errorcluster, "handle out"=w62:i16)  [unwired: 4 in]
    n13 = call "PicoScope6000aGetValuesOverlapped.vi"("Segment Range"="Segment Range", "Buffer and Transfer Settings"="Buffer and Transfer Settings", "error in (no error)"=w63, "handle in"=w62) -> ("error out"=w45:errorcluster, "handle out"=w44:i16, "Pointer to Overflow"=w33:u64[], "noOfSamples"=w24:u64)  [unwired: 4 in]
    n14 = call "PicoScope6000aGetTimebase2.vi"("Number of Samples"=w24, "Acquisition Settings"="Acquisition Settings", "error in (no error)"=w45, "handle in"=w44) -> ("error out"=w52:errorcluster, "handle out"=w53:i16, "Properties Panel"=w56:T7)  [unwired: 5 in]
    "Properties Panel" <- w56
    n15 = Unbundle By Name(w34) -> ("PICO_VARIANT_INFO"=w35:string)
    n16 = call "PicoScope6000aRunBlock.vi"("Acquisition Settings"="Acquisition Settings", "error in (no error)"=w52, "handle in"=w53) -> ("error out"=w51:errorcluster, "handle out"=w50:i16)  [unwired: 5 in, 2 out]
    n17 = while {
      shift-right: [w155] -> w39
      shift-left: w51 -> [w156]
      shift-right: [w154] -> w36
      shift-left: w50 -> [w153]
      stop <- w151 stop-if-true
      n18 = call "PicoScope6000aIsReady.vi"("error in (no error)"=w156, "handle in"=w153) -> ("error out"=w155:errorcluster, "handle out"=w154:i16, "ready"=w152:i16)  [unwired: 7 in]
      n19 = Not Equal To 0?(x=w152) -> (x != 0?=w150:bool)
      n20 = Or(x=w150, y="stop") -> (x .or. y?=w151:bool)
      n21 = Wait (ms)(milliseconds to wait=u32 10) -> ()  [unwired: 1 out]
    }
    n22 = Unbundle By Name(w56) -> ("Sample Rate"=w41:dbl)
    n23 = call "PicoScope6000aStop.vi"("error in (no error)"=w39, "handle in"=w36) -> ("error out"=w38:errorcluster, "handle out"=w37:i16)  [unwired: 8 in]
    n24 = Unbundle By Name("Segment Range") -> ("toSegmentIndex"=w29:u64, "fromSegmentIndex"=w28:u64)
    n25 = call "PicoScope6000aGetTriggerInfo.vi"("handle in"=w37, "Segment Range"="Segment Range", "Sample Rate"=w41, "error in"=w38) -> ("handle out"=w42:i16, "Trigger Offsets"=→"Trigger Offsets":cluster{"Samples":u64, "Time (seconds)":sgl}[], "error out"=w43:errorcluster)  [unwired: 8 in, 1 out]
    n26 = call "PicoReadPicoMultiBuffers.vi"("enabled array"=w71, "Buffer and Transfer Settings"="Buffer and Transfer Settings", "Variant"=w35, "Data Pointers"=w70, "No of Buffers"=w60, "error in (no error)"=w43) -> ("MultiBuffers (Max or non-aggregated)"=w59:T11, "error out"=w49:errorcluster)  [unwired: 7 in, 1 out]
    n27 = Subtract(x=w29, y=w28) -> (x-y=w30:u64)
    n28 = Unbundle By Name("Buffer and Transfer Settings") -> ("Down-Sample Mode"=w57:u32, "Down Sample Ratio"=w58:u64)
    n29 = case shown="80000000" w57 {
      tunnel: [w157 u64 1 ("Down Sample Ratio")] -> w54
      tunnel: w58 -> [w157 _]
      frame Default {
      }
      frame -2147483648 {
        # "No DownSampling"
      }
    }
    n30 = Multiply(x=w54, y=w41) -> (x*y=w55:dbl)
    n31 = while {
      tunnel: w78 -> [w147]
      tunnel: "Channels" -> [w146]
      tunnel: w59 -> [w96]
      tunnel: w55 -> [w95]
      shift-right: [w145] -> w69
      shift-left: w68 -> [w144]
      tunnel: [w85] -> w25
      tunnel: w49 -> [w86]
      tunnel: ["Stop Display"] -> w48
      tunnel: w33 -> [w81]
      tunnel: w30 -> [w82]
      tunnel: [w81] -> w27
      stop <- w89 stop-if-true
      w104 = u16 0 items=["unsigned binary", "offset binary", "2's complement"] ("data format (offset binary)")
      n32 = Index Array(array=w96, index="Display Buffer Index") -> (element=w94:T12)
      n33 = Unbundle By Name(w94) -> ("Channel H Buffer"=w102:i16[])
      n34 = Unbundle By Name(w146) -> ("Channel H Settings.Range"=w124:u16)
      n35 = Unbundle By Name(w146) -> ("Channel G Settings.Range"=w125:u16)
      n36 = Unbundle By Name(w94) -> ("Channel G Buffer"=w126:i16[])
      n37 = Unbundle By Name(w146) -> ("Channel D Settings.Range"=w131:u16)
      n38 = Unbundle By Name(w94) -> ("Channel E Buffer"=w130:i16[])
      n39 = Unbundle By Name(w146) -> ("Channel E Settings.Range"=w129:u16)
      n40 = Unbundle By Name(w94) -> ("Channel F Buffer"=w128:i16[])
      n41 = Unbundle By Name(w146) -> ("Channel F Settings.Range"=w127:u16)
      n42 = Unbundle By Name(w94) -> ("Channel A Buffer"=w93:i16[])
      n43 = Unbundle By Name(w146) -> ("Channel A Settings.Range"=w142:u16)
      n44 = Unbundle By Name(w94) -> ("Channel D Buffer"=w132:i16[])
      n45 = Unbundle By Name(w94) -> ("Channel B Buffer"=w140:i16[])
      n46 = Unbundle By Name(w146) -> ("Channel B Settings.Range"=w139:u16)
      n47 = Unbundle By Name(w94) -> ("Channel C Buffer"=w134:i16[])
      n48 = Unbundle By Name(w146) -> ("Channel C Settings.Range"=w133:u16)
      n49 = Unbundle By Name(w94) -> ("Port 0 Buffer"=w101:i16[])
      n50 = To Long Integer(number=w82) -> (32bit integer=w83:i32)
      n51 = call "PicoScopeAdcToVolts.vi"("Max_adc"=w147, "Range Index"=w124, "Data"=w102) -> ("Data"=w119:dbl[])
      n52 = call "PicoScopeAdcToVolts.vi"("Max_adc"=w147, "Range Index"=w142, "Data"=w93) -> ("Data"=w97:dbl[])
      n53 = call "PicoScopeAdcToVolts.vi"("Max_adc"=w147, "Range Index"=w125, "Data"=w126) -> ("Data"=w113:dbl[])
      n54 = call "PicoScopeAdcToVolts.vi"("Max_adc"=w147, "Range Index"=w129, "Data"=w130) -> ("Data"=w116:dbl[])
      n55 = call "PicoScopeAdcToVolts.vi"("Max_adc"=w147, "Range Index"=w127, "Data"=w128) -> ("Data"=w112:dbl[])
      n56 = call "PicoScopeAdcToVolts.vi"("Max_adc"=w147, "Range Index"=w131, "Data"=w132) -> ("Data"=w117:dbl[])
      n57 = call "PicoScopeAdcToVolts.vi"("Max_adc"=w147, "Range Index"=w139, "Data"=w140) -> ("Data"=w138:dbl[])
      n58 = call "PicoScopeAdcToVolts.vi"("Max_adc"=w147, "Range Index"=w133, "Data"=w134) -> ("Data"=w118:dbl[])
      n59 = call "ReadBuffer.vi"("Pointer and BufferSize"=w81, "Buffer size"=w83, "error in (no error)"=w86) -> ("Output Array"=→"overflow":i16[], "error out"=w85:errorcluster)  [unwired: 11 in]
      n60 = TDMS Write(0:w144, 9:w93) -> (4:w145:refnum<k34>)  [unwired: 4 in, 3 out]
      n61 = Bundle(0, w95, "Data"=w97) -> (w137:cluster{i32, dbl, "Data":dbl[]})  [unwired: 1 in]
      n62 = Bundle(0, w95, "Data"=w138) -> (w136:cluster{i32, dbl, "Data":dbl[]})  [unwired: 1 in]
      n63 = Bundle(0, w95, "Data"=w118) -> (w111:cluster{i32, dbl, "Data":dbl[]})  [unwired: 1 in]
      n64 = Bundle(0, w95, "Data"=w116) -> (w109:cluster{i32, dbl, "Data":dbl[]})  [unwired: 1 in]
      n65 = Bundle(0, w95, "Data"=w112) -> (w108:cluster{i32, dbl, "Data":dbl[]})  [unwired: 1 in]
      n66 = Bundle(0, w95, "Data"=w113) -> (w107:cluster{i32, dbl, "Data":dbl[]})  [unwired: 1 in]
      n67 = Bundle(0, w95, "Data"=w117) -> (w110:cluster{i32, dbl, "Data":dbl[]})  [unwired: 1 in]
      n68 = Bundle(0, w95, "Data"=w119) -> (w106:cluster{i32, dbl, "Data":dbl[]})  [unwired: 1 in]
      n69 = call-poly <vilib>:"Analog to Digital.vi"("data format (offset binary)"=w104, "full-scale range (pk-pk)"=256.0, "resolution (16 bit)"=8, "analog waveform"=w101) -> ("digital waveform"=w98:digitalwaveform)  [unwired: 4 in, 3 out]
      n70 = Or(x="Stop Display", y="Run") -> (x .or. y?=w89:bool)
      n71 = local write "Capture Complete"(TRUE ("Capture Complete")) -> ()
      n72 = Build Array(w137, w136, w111, w110, w109, w108, w107, w106) -> (→"Analog Channels":cluster{i32, dbl, "Data":dbl[]}[])
      n73 = Bundle By Name("t0"=timestamp(0 s since 1904-01-01), "dt"=w95, "Y"=w98) -> (→"Port 0":digitalwaveform)  [unwired: 1 in]
      n74 = Wait (ms)(milliseconds to wait=u32 100) -> ()  [unwired: 1 out]
    }
    n75 = call "ReleaseBuffer.vi"("error in (no error)"=w25, "Pointer and BufferSize"=w27) -> ("error out"=w26:errorcluster)  [unwired: 9 in]
    "Capture Complete" <- FALSE ("Capture Complete")
  }
  n76 = TDMS Close(11:w3) -> ()  [unwired: 1 in, 2 out]
  n77 = call "PicoScope6000aClose.vi"("error in (no error)"=w12, "handle in"=w11) -> ("error out"=w10:errorcluster)  [unwired: 8 in, 1 out]
  n78 = call "PicoReleaseMultiBuffers.vi"("error in (no error)"=w10, "Enabled array"=w14, "Data Pointers"=w13) -> ("error out"=→"error out":errorcluster)  [unwired: 8 in]
